vi "Init.Pub.vi"(1 "MQTT":cluster{"address (IP)":string, "port":u16}={"address (IP)"="127.0.0.1", "port"=1883}, 2 "ZMQ":string="tcp://*:5000") -> (0 "Pub":T1)   [LabVIEW 2014]
uses:
  <vilib>/addons/zeromq/zmq_socket.lvclass
  <vilib>/addons/zeromq/zmq_context.lvclass
  <vilib>/addons/zeromq/socket_type.ctl
  <vilib>/daq.io/MQTT LabVIEW Client/Controls/Connect_Flags.ctl
  <vilib>/daq.io/MQTT LabVIEW Client/Controls/QoS.ctl
  <vilib>/daq.io/MQTT LabVIEW Client/Controls/DUP_Flag.ctl
  <vilib>/daq.io/MQTT LabVIEW Client/Controls/Retain_Flag.ctl
  Pub.global.vi
  <vilib>/daq.io/MQTT LabVIEW Client/MQTT_Functions.lvlib
  <vilib>/addons/zeromq/zeromq.lvlib
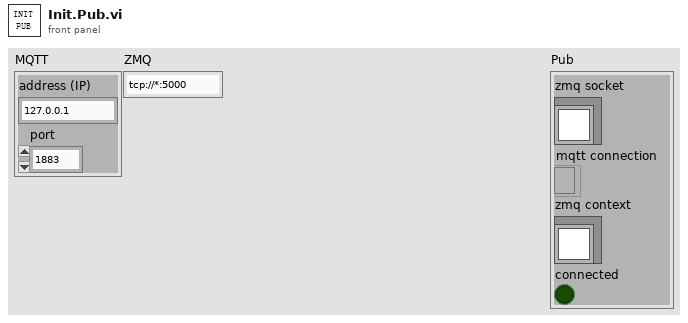
[diagram p1: front panel]
types:
  T1 = cluster{"zmq socket":refnum<class "zmq_socket.lvclass">, "mqtt connection":refnum<k5>, "zmq context":refnum<class "zmq_context.lvclass">, "connected":bool}
  T2 = typedef "MQTT_Functions.lvlib/QoS.ctl" = enum8{"At most once", "At least once", "Exactly once", "Reserved"}
  T3 = typedef "MQTT_Functions.lvlib/DUP_Flag.ctl" = bool
  T4 = typedef "MQTT_Functions.lvlib/Retain_Flag.ctl" = bool
  T5 = cluster{"QoS":T2, "DUP":T3, "Retain":T4, "Keep Alive (sec)":u16}
  T6 = typedef "MQTT_Functions.lvlib/Connect_Flags.ctl" = cluster{"user name":bool, "password":bool, "will retain":bool, "will flag":bool, "clean session":bool, "reserved":bool, "will QoS":T2}
  T7 = typedef "zeromq.lvlib/socket_type.ctl" = enum8{"ZMQ_PAIR", "ZMQ_PUB", "ZMQ_SUB", "ZMQ_REQ", "ZMQ_REP", "ZMQ_DEALER", "ZMQ_ROUTER", "ZMQ_PULL", "ZMQ_PUSH", "ZMQ_XPUB", "ZMQ_XSUB"}
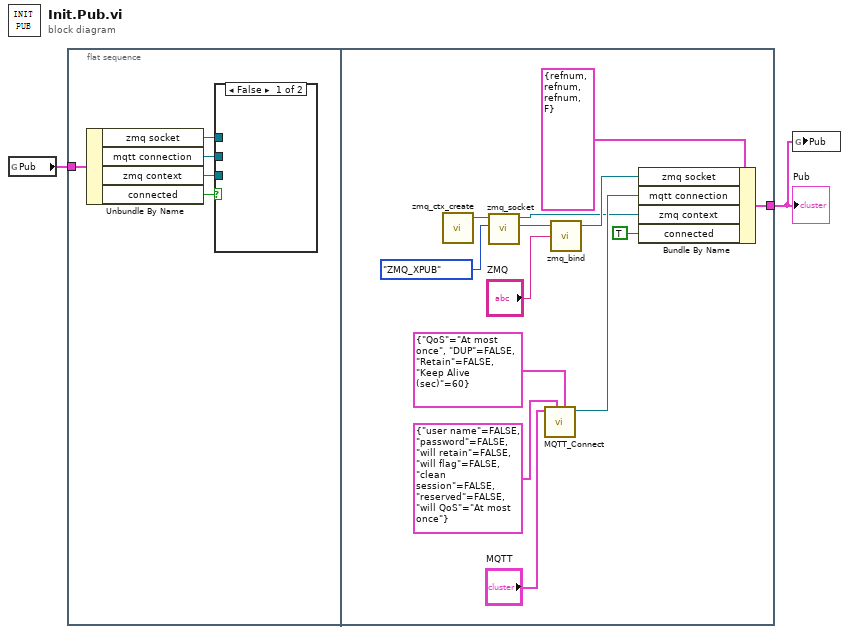
[diagram p0: block diagram]
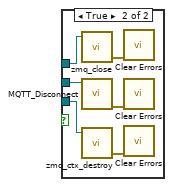
[diagram p2: hidden frame]
diagram:
  n1 = global read "Pub.global.vi" "Pub"() -> (w2:T1)
  n2 = flat-sequence {
    tunnel: w2 -> [w7]
    tunnel: [w14] -> w1
    frame #0 {
      n3 = Unbundle By Name(w7) -> ("zmq socket"=w5:refnum<class "zmq_socket.lvclass">, "mqtt connection"=w3:refnum<k5>, "zmq context"=w4:refnum<class "zmq_context.lvclass">, "connected"=w6:bool)
      n4 = case shown="False" w6 {
        tunnel: w5 -> [_ w11]
        tunnel: w4 -> [_ w10]
        tunnel: w3 -> [_ w13]
        frame False {
        }
        frame True {
          n5 = call <vilib>:"zmq_close.vi"("socket"=w11) -> ("error out"=w9:errorcluster)  [unwired: 4 in]
          n6 = call <vilib>:"MQTT_Disconnect.vi"("connection ID"=w13) -> ("error out"=w12:errorcluster)  [unwired: 10 in]
          n7 = call <vilib>:"zmq_ctx_destroy.vi"("context in"=w10) -> ("error out"=w8:errorcluster)  [unwired: 4 in]
          n8 = call <vilib>:"Clear Errors.vi"("error in (no error)"=w9) -> ()  [unwired: 5 in, 2 out]
          n9 = call <vilib>:"Clear Errors.vi"("error in (no error)"=w12) -> ()  [unwired: 5 in, 2 out]
          n10 = call <vilib>:"Clear Errors.vi"("error in (no error)"=w8) -> ()  [unwired: 5 in, 2 out]
        }
      }
    }
    frame #1 {
      n11 = call <vilib>:"zmq_ctx_create.vi"() -> ("context out"=w24:refnum<class "zmq_context.lvclass">)  [unwired: 4 in, 1 out]
      n12 = call <vilib>:"zmq_socket.vi"("socket type"=socket_type."ZMQ_XPUB", "context in"=w24) -> ("socket out"=w20:refnum<class "zmq_socket.lvclass">, "context out"=w15:refnum<class "zmq_context.lvclass">)  [unwired: 3 in, 1 out]
      n13 = call <vilib>:"MQTT_Connect.vi"("Connect Meta"=T5 {"QoS"=enum."At most once", "DUP"=FALSE, "Retain"=FALSE, "Keep Alive (sec)"=60}, "Connect Flags"=T6 {"user name"=FALSE, "password"=FALSE, "will retain"=FALSE, "will flag"=FALSE, "clean session"=FALSE, "reserved"=FALSE, "will QoS"=enum."At most once"}, "MQTT Broker"="MQTT") -> ("connection ID out"=w17:refnum<k5>)  [unwired: 6 in, 2 out]
      n14 = call <vilib>:"zmq_bind.vi"("endpoint"="ZMQ", "socket in"=w20) -> ("socket out"=w16:refnum<class "zmq_socket.lvclass">)  [unwired: 2 in, 1 out]
      n15 = Bundle By Name(cluster=T1 {"zmq socket"=refnum, "mqtt connection"=refnum, "zmq context"=refnum, "connected"=FALSE} ("Pub"), "zmq socket"=w16, "mqtt connection"=w17, "zmq context"=w15, "connected"=TRUE) -> (w14:T1)
    }
  }
  n16 = global write "Pub.global.vi" "Pub"(w1) -> ()
  "Pub" <- w1
